vi "sync publish timing.vi"(8 "error in (no error)":errorcluster, 10 "parameters data in":T1, 11 "module in":refnum<class "Shared Memory runtime.lvclass">) -> (0 "error out":errorcluster, 2 "parameters data out":T1, 3 "module out":refnum<class "Shared Memory runtime.lvclass">)   [LabVIEW 2014, in "Shared Memory runtime.lvclass"]
uses:
  Shared Memory runtime.lvclass
  <vilib>/NI/Tag Bus/table/data table.ctl
  Shared Memory runtime.lvclass/Shared Memory runtime.ctl
  <vilib>/NI/NI Linux RT IPC/Shared Memory/Pointer Operations/Write Scalar I64.vi
  <vilib>/NI/Tag Bus/table/data polymorphs/read one/read Double.vi
  <vilib>/NI/NI Linux RT IPC/POSIX Threads/Classes/Semaphore/Semaphore.lvclass
  <vilib>/NI/NI Linux RT IPC/Shared Memory/Classes/Shared Memory/Shared Memory.lvclass
  <vilib>/NI/NI Linux RT IPC/Shared Memory/Shared Memory.lvlib
  <vilib>/NI/Tag Bus/table/data table.lvlib
  <vilib>/NI/NI Linux RT Utilities/Linux RT Utilities.lvlib
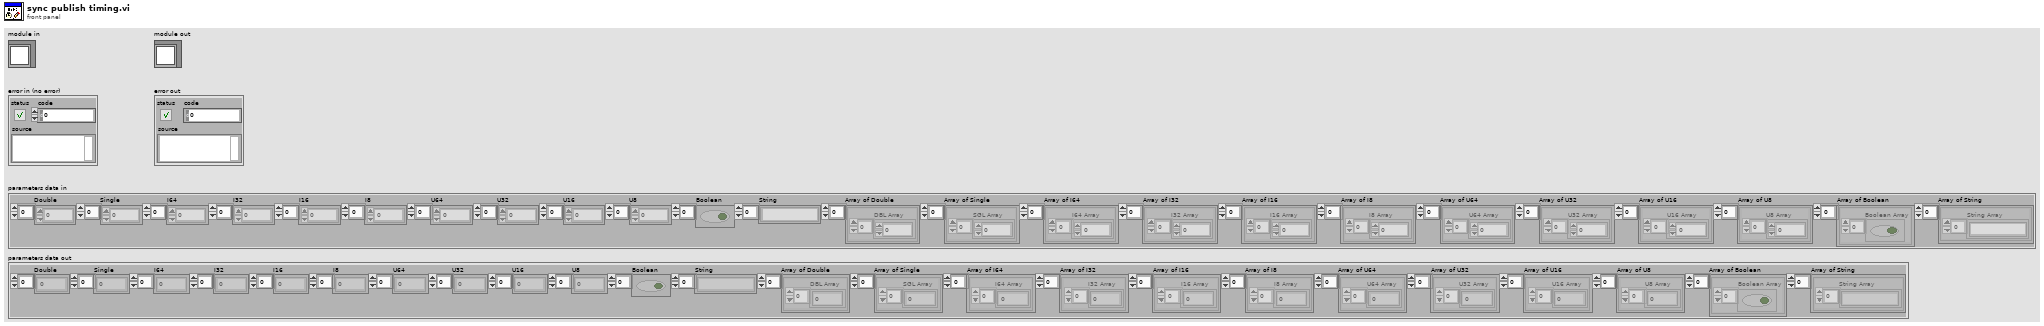
[diagram p1: front panel]
types:
  T1 = typedef "tag bus.lvlib/data table.lvlib/data table.ctl" = cluster{"Double":dbl[], "Single":sgl[], "I64":i64[], "I32":i32[], "I16":i16[], "I8":i8[], "U64":u64[], "U32":u32[], "U16":u16[], "U8":u8[], "Boolean":bool[], "String":string[], "Array of Double":cluster{"DBL Array":dbl[]}[], "Array of Single":cluster{"SGL Array":sgl[]}[], "Array of I64":cluster{"I64 Array":i64[]}[], "Array of I32":cluster{"I32 Array":i32[]}[], "Array of I16":cluster{"I16 Array":i16[]}[], "Array of I8":cluster{"I8 Array":i8[]}[], "Array of U64":cluster{"U64 Array":u64[]}[], "Array of U32":cluster{"U32 Array":u32[]}[], "Array of U16":cluster{"U16 Array":u16[]}[], "Array of U8":cluster{"U8 Array":u8[]}[], "Array of Boolean":cluster{"Boolean Array":bool[]}[], "Array of String":cluster{"String Array":string[]}[]}
  T2 = typedef "Shared Memory runtime.lvclass/sync data.ctl" = cluster{"semaphores soc":T3[], "semaphores eoc":T3[], "timeout":dbl, "enabled":bool, "sync shared memory":T5, "publish timing":bool, "timing indices":T6, "timing pointers":T7}
  T3 = typedef "Shared Memory runtime.lvclass/semaphore data.ctl" = cluster{"semaphore":T4, "name":string}
  T4 = typedef "Linux RT IPC.lvlib/POSIX Threads.lvlib/Semaphore.lvclass/reference.ctl" = refnum<data-value>
  T5 = typedef "Linux RT IPC.lvlib/Shared Memory.lvlib/reference.ctl" = refnum<data-value>
  T6 = typedef "Shared Memory runtime.lvclass/sync timing indices.ctl" = cluster{"start time index":i32}
  T7 = typedef "Shared Memory runtime.lvclass/sync timing pointers.ctl" = cluster{"start sec ptr":u64, "start nsec ptr":u64}
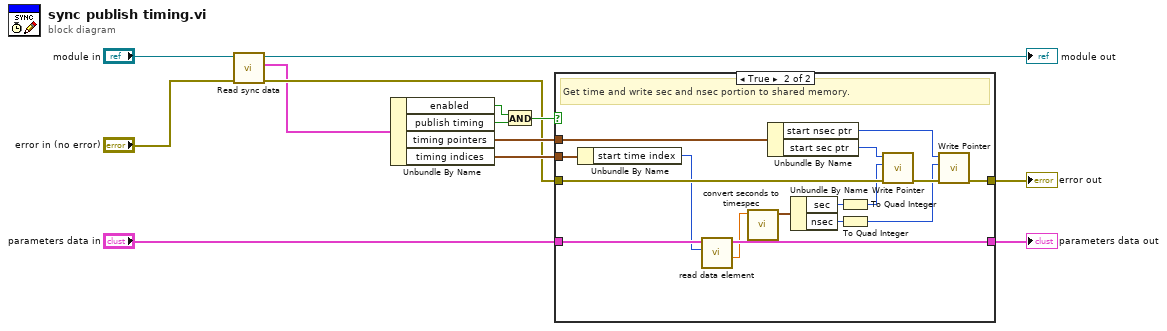
[diagram p0: block diagram]
diagram:
  n1 = call "Read sync data.vi"("error in (no error)"="error in (no error)", "Shared Memory runtime in"="module in") -> ("error out"=w2:errorcluster, "sync data"=w1:T2, "Shared Memory runtime out"=→"module out":refnum<class "Shared Memory runtime.lvclass">)  [unwired: 7 in]
  n2 = Unbundle By Name(w1) -> ("enabled"=w7:bool, "publish timing"=w8:bool, "timing pointers"=w13:T7, "timing indices"=w11:T6)
  n3 = And(x=w7, y=w8) -> (x .and. y?=w6:bool)
  n4 = case shown="True" w6 {
    tunnel: w2 -> [w15 w31]
    tunnel: w13 -> [_ w28]
    tunnel: [w15 w29] -> w12
    tunnel: w11 -> [_ w25]
    tunnel: "parameters data in" -> [w14 w24]
    tunnel: [w14 w23] -> w9
    frame False {
      # "Not enabled, so do nothing."
    }
    frame True {
      # "Get time and write sec and nsec portion to shared memory."
      n5 = Unbundle By Name(w25) -> ("start time index"=w22:i32)
      n6 = call-poly <vilib>:"read data element.vi"("index"=w22, "data table in"=w24) -> ("value"=w21:dbl, "data table out"=w23:T1)  [unwired: 8 in]
      n7 = call <vilib>:"convert seconds to timespec.vi"("seconds"=w21) -> ("timespec"=w20:cluster{"sec":u64, "nsec":u64})  [unwired: 10 in]
      n8 = Unbundle By Name(w28) -> ("start nsec ptr"=w27:u64, "start sec ptr"=w26:u64)
      n9 = Unbundle By Name(w20) -> ("sec"=w19:u64, "nsec"=w18:u64)
      n10 = To Quad Integer(1:w19) -> (0:w17:i64)
      n11 = To Quad Integer(1:w18) -> (0:w16:i64)
      n12 = call-poly <vilib>:"Write Pointer.vi"("error in (no error)"=w31, "value"=w17, "pointer in"=w26) -> ("error out"=w30:errorcluster)  [unwired: 7 in, 1 out]
      n13 = call-poly <vilib>:"Write Pointer.vi"("error in (no error)"=w30, "value"=w16, "pointer in"=w27) -> ("error out"=w29:errorcluster)  [unwired: 7 in, 1 out]
    }
  }
  "error out" <- w12
  "parameters data out" <- w9
